vi "Client Loops.vi"(11 "TCPMessaging in":refnum<class "TCPMessaging.lvclass">) -> ()   [LabVIEW 2020, in "Vecto.lvlib" / "TCPMessaging.lvclass"]
uses:
  TCPMessaging.lvclass
  TCPMessaging.lvclass/TCPMessaging.ctl
panel:
  out "node_alias":string
  out "node_name":string
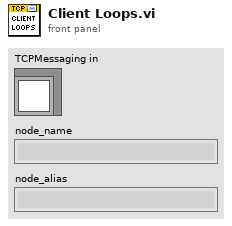
[diagram p1: front panel]
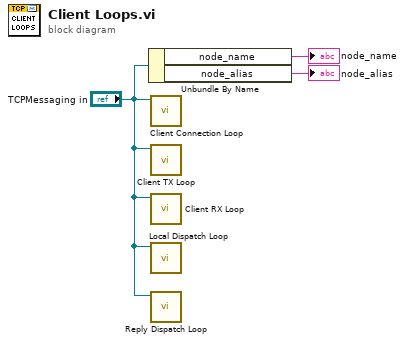
[diagram p0: block diagram]
diagram:
  n1 = Unbundle By Name("TCPMessaging in") -> ("node_name"=→"node_name":string, "node_alias"=→"node_alias":string)
  n2 = call "Client Connection Loop.vi"("TCPMessaging in"="TCPMessaging in") -> ()  [unwired: 10 in, 1 out]
  n3 = call "Client TX Loop.vi"("TCPMessaging in"="TCPMessaging in") -> ()  [unwired: 10 in, 1 out]
  n4 = call "Client RX Loop.vi"("TCPMessaging in"="TCPMessaging in") -> ()  [unwired: 10 in, 1 out]
  n5 = call "Local Dispatch Loop.vi"("TCPMessaging in"="TCPMessaging in") -> ()  [unwired: 11 in]
  n6 = call "Reply Dispatch Loop.vi"("TCPMessaging in"="TCPMessaging in") -> ()  [unwired: 10 in, 1 out]
